vi "Versioned Load AQT.vi"(11 "Path":path) -> (3 "data":T5)   [LabVIEW 2025]
uses:
  Types/Decision Tree.ctl
  Types/Sequencing Tree Node.ctl
  Types/Single Cmd Info.ctl
  <vilib>/picture/picture.llb/imagedata.ctl
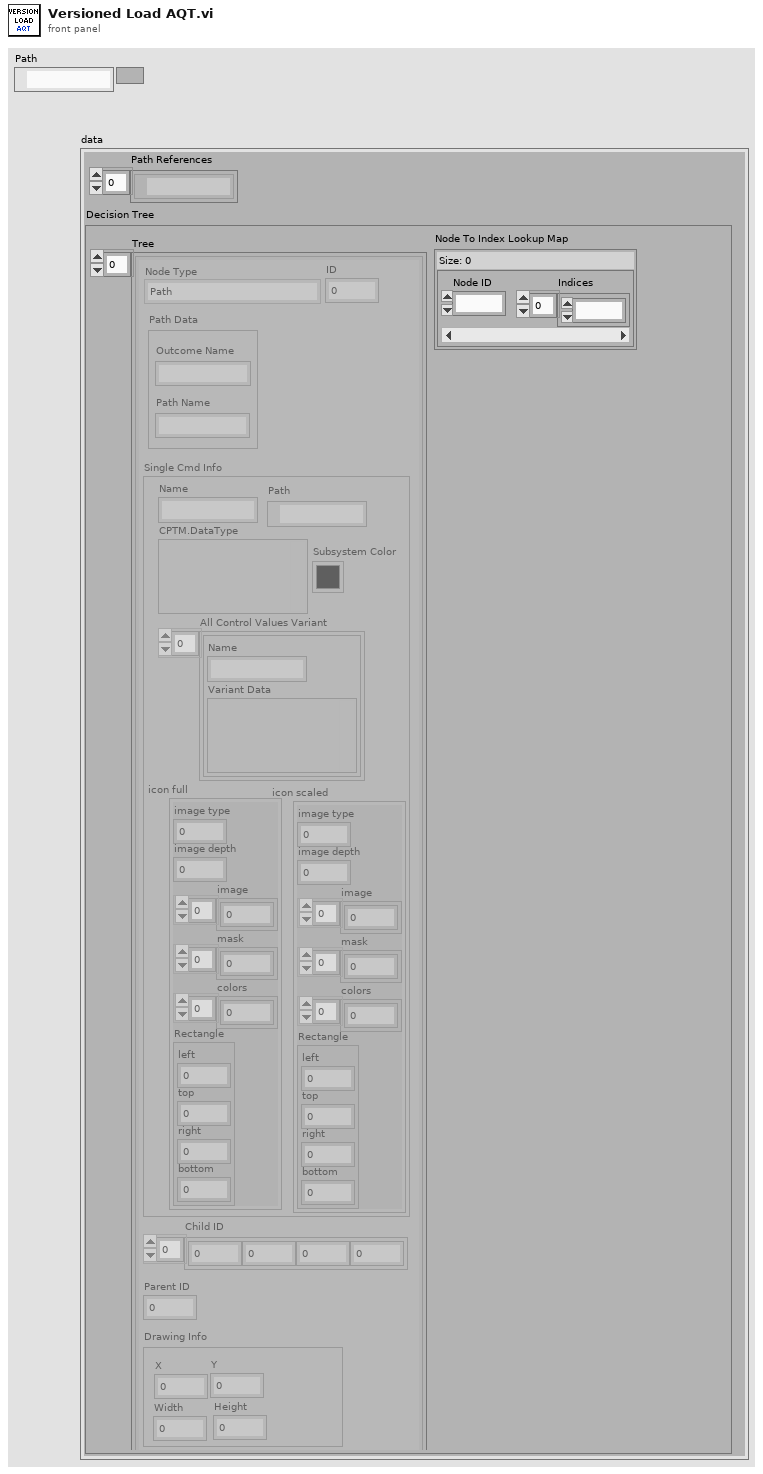
[diagram p1: front panel]
types:
  T1 = typedef "Decision Tree.ctl" = cluster{"Tree":T2[], "Node To Index Lookup Map":map{i16, i16[]}}
  T2 = typedef "Sequencing Tree Node.ctl" = cluster{"Node Type":enum16{"Path", "Command", "Leaf"}, "ID":i16, "Path Data":cluster{"Path Name":string, "Outcome Name":string}, "Single Cmd Info":T3, "Child ID":i32[], "Parent ID":i32, "Drawing Info":cluster{"X":i32, "Y":i32, "Width":i32, "Height":i32}}
  T3 = typedef "Single Cmd Info.ctl" = cluster{"Name":string, "CPTM.DataType":variant, "All Control Values Variant":cluster{"Name":string, "Variant Data":variant}[], "icon full":T4, "icon scaled":T4, "Path":path, "Subsystem Color":u32}
  T4 = typedef "imagedata.ctl" = cluster{"image type":i32, "image depth":i32, "image":u8[], "mask":u8[], "colors":u32[], "Rectangle":cluster{"left":i16, "top":i16, "right":i16, "bottom":i16}}
  T5 = cluster{"Path References":path[], "Decision Tree":T1}
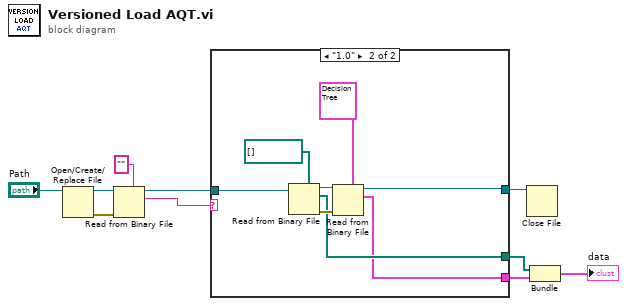
[diagram p0: block diagram]
diagram:
  n1 = Open/Create/Replace File(file path (use dialog)="Path") -> (refnum out=w8:refnum<file>, error out=w9:errorcluster)  [unwired: 5 in, 1 out]
  n2 = Read from Binary File(5:"", 8:w9, 11:w8) -> (2:w6:string, 3:w5:refnum<file>)  [unwired: 3 in, 2 out]
  n3 = case shown="\"1.0\"" w6 {
    tunnel: w5 -> [w11 w18]
    tunnel: [_ w15] -> w4
    tunnel: [w11 w14] -> w3
    tunnel: [_ w12] -> w2
    frame "False", Default {
    }
    frame "1.0" {
      n4 = Read from Binary File(5:path[] [] ("Path Reference"), 11:w18) -> (0:w19:errorcluster, 2:w15:path[], 3:w17:refnum<file>)  [unwired: 4 in, 1 out]
      n5 = Read from Binary File(5:T1 data[7007B], 8:w19, 11:w17) -> (2:w12:T1, 3:w14:refnum<file>)  [unwired: 3 in, 2 out]
    }
  }
  n6 = Close File(refnum=w3) -> ()  [unwired: 1 in, 2 out]
  n7 = Bundle("Path Reference"=w4, w2) -> (→"data":cluster{"Path Reference":path[], T1})  [unwired: 1 in]
